vi "Main.vi"() -> ()   [LabVIEW 2021]
doc: "Use this template to build a simple state machine design pattern. Each state executes code and determines which state to transition to."
uses:
  controls/State.ctl
  controls/Data.ctl
  vmmso/vmmso.lvlib
panel:
  out "IO Read Return":u32 format="%x"
  out "IO4":bool
  out "IO0":bool
  out "Is IO Ready?":bool
  in  "DDS2 Amplitude":dbl=2000.0
  in  "DDS2 Bias":dbl
  in  "DDS2 Freq":dbl=1000.0
  in  "DDS2 Wave Style":u16(ring) items=["Sine", "Square", "Ramp"]
  in  "DDS1 Amplitude":dbl=2000.0
  in  "DDS1 Bias":dbl
  in  "DDS1 Freq":dbl=1000.0
  in  "DDS1 Wave Style":u16(ring) items=["Sine", "Square", "Ramp"]
  out "Is Data Ready？":bool
  out "ReadVoltageData Return":u32
  out "Voltage Wave":dbl[][](graph)
  out "Capture Return":i32
  out "Device is OK?":bool
  out "Support Samples":u32[](array[numeric])
  in  "Exit":bool
  # "DDS1"
  # "DDS2"
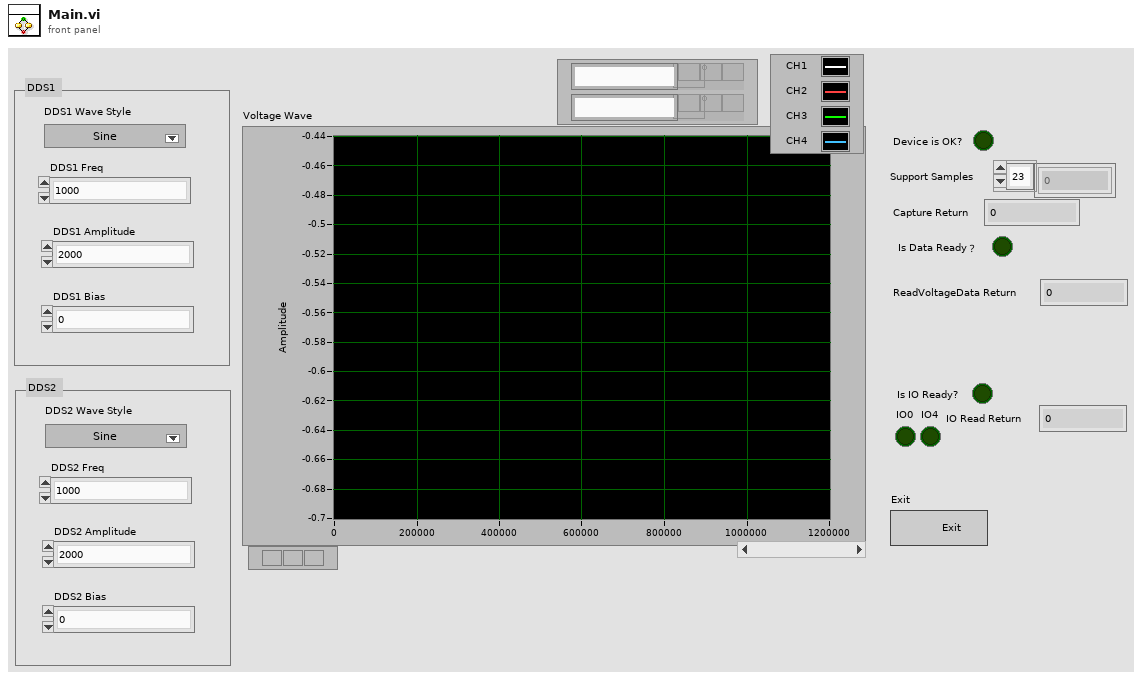
[diagram p1: front panel]
types:
  T1 = typedef "Data.ctl" = cluster{"Boolean <Is Exit>":bool, "String <Replace Me>":string, "Numeric <Replace Me>":dbl}
  T2 = typedef "State.ctl" = enum16{"Initialize", "Wait for UsbIn", "Init Osc and Dds", "Wait for Event", "Capture", "Read Voltage", "Read IO", "Exit"}
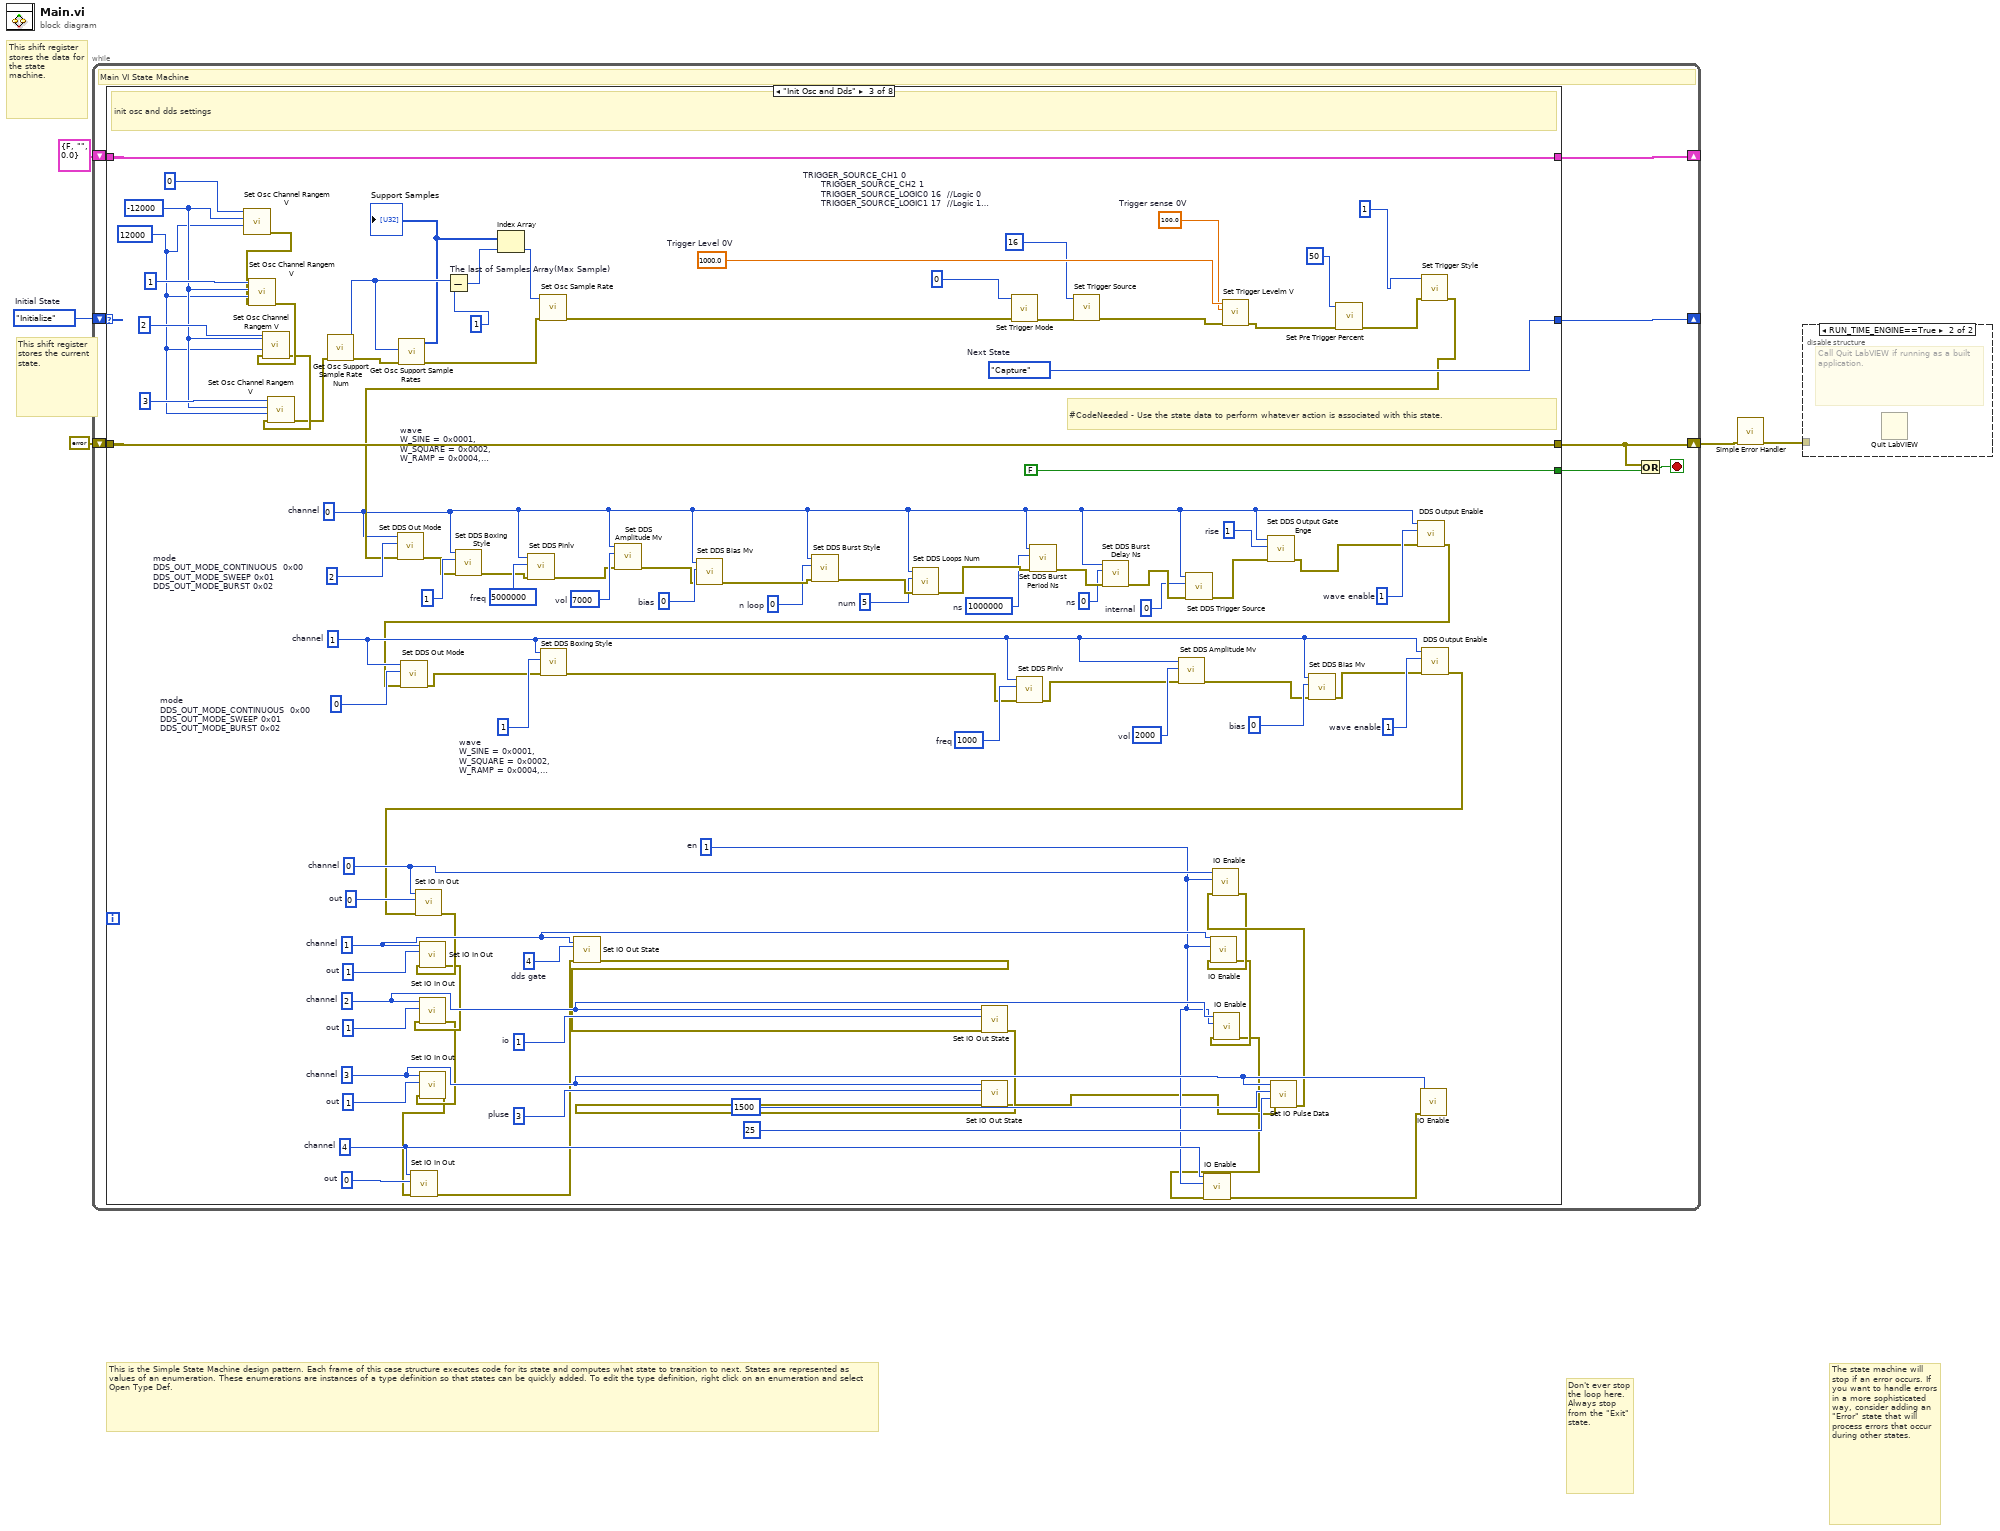
[diagram p0: block diagram]
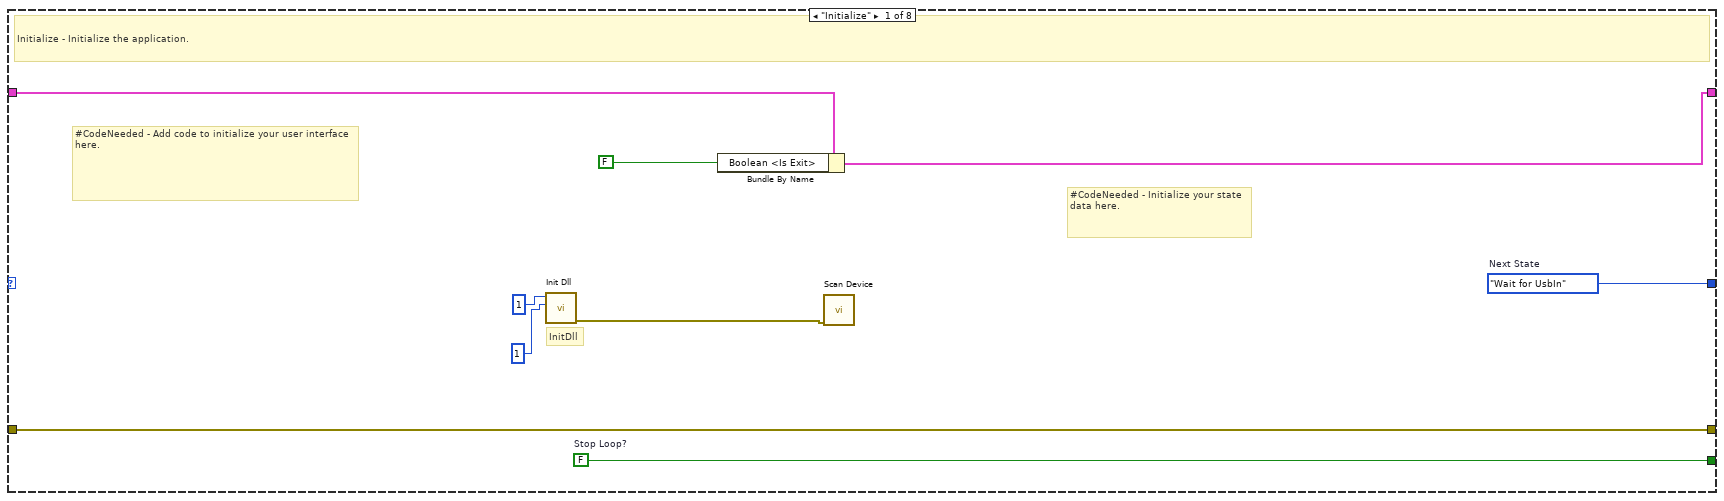
[diagram p3: hidden frame]
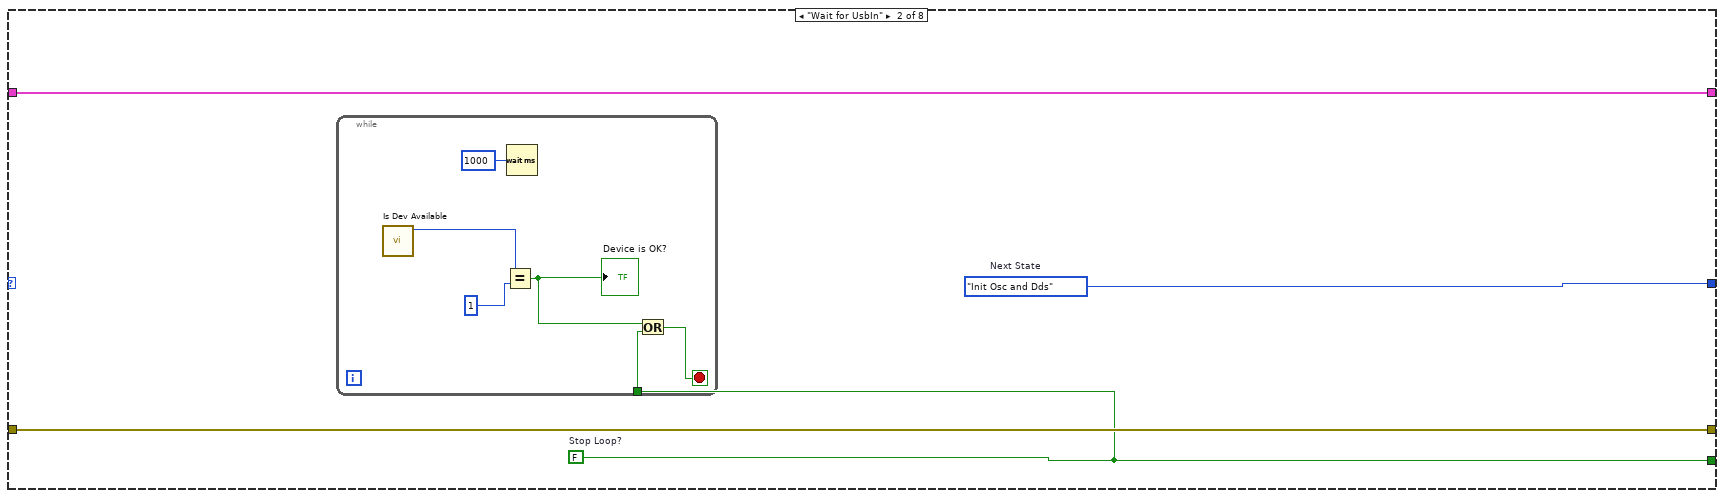
[diagram p4: hidden frame]
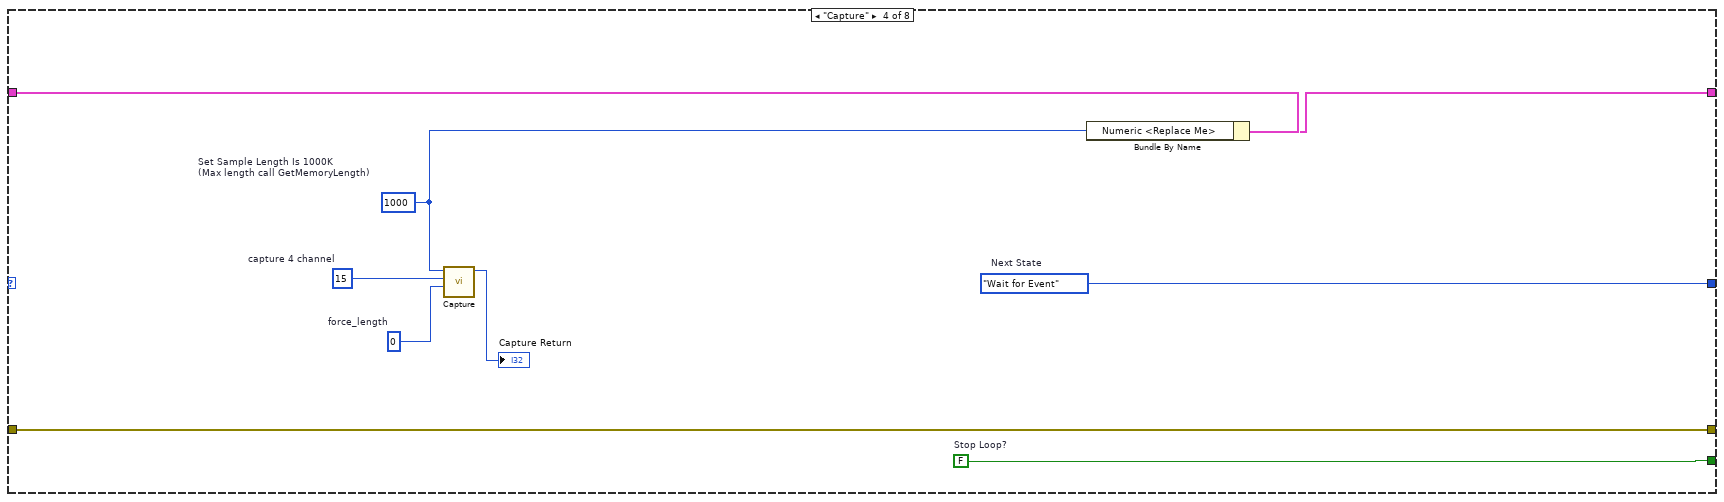
[diagram p5: hidden frame]
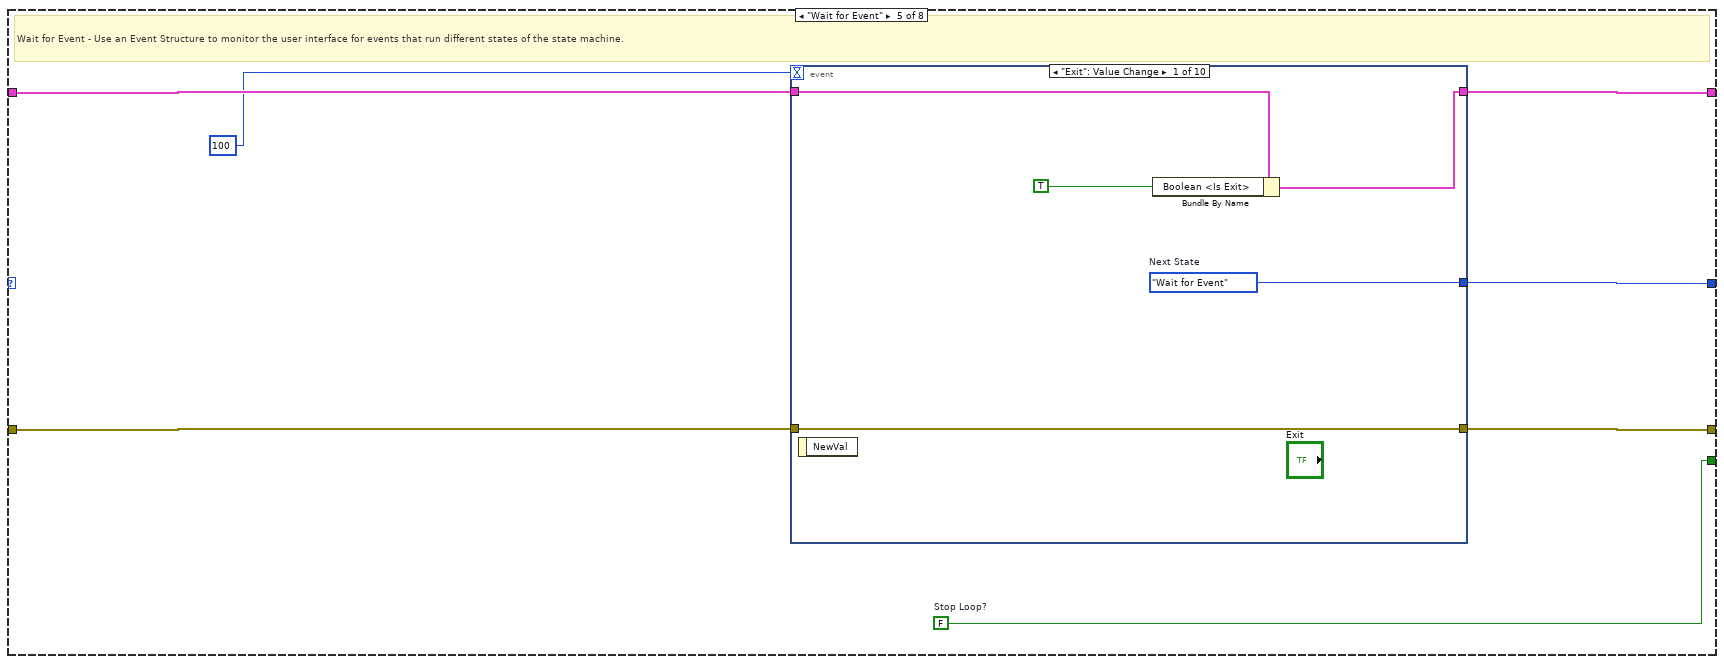
[diagram p6: hidden frame]
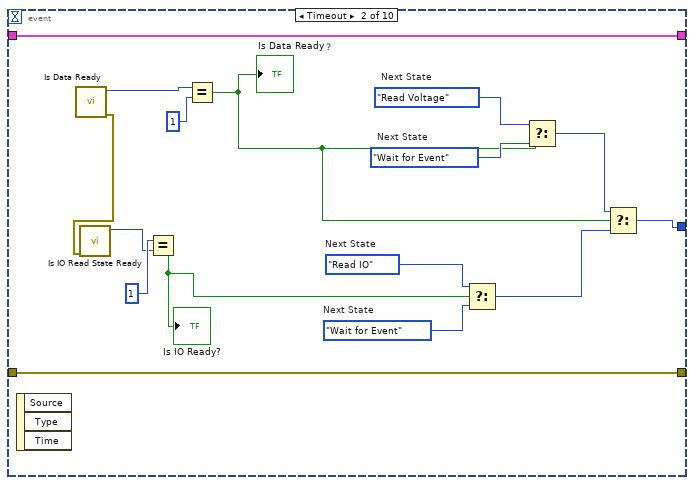
[diagram p7: hidden frame]
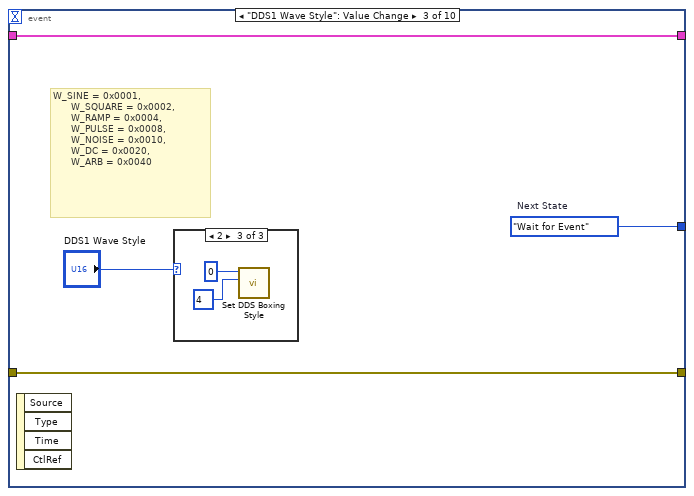
[diagram p8: hidden frame]
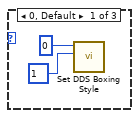
[diagram p9: hidden frame]
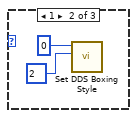
[diagram p10: hidden frame]
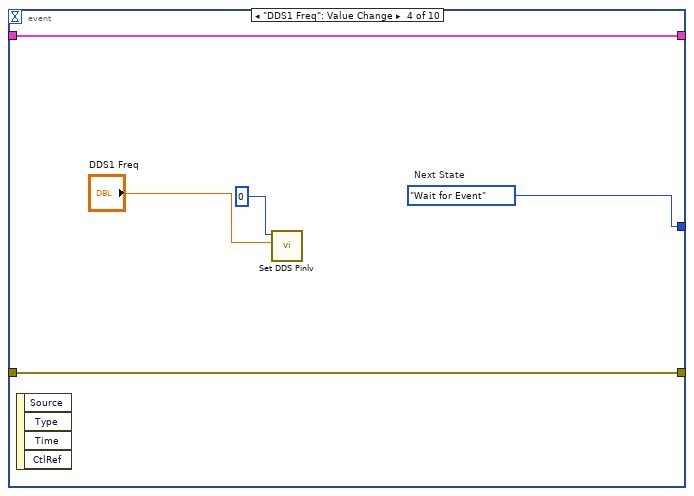
[diagram p11: hidden frame]
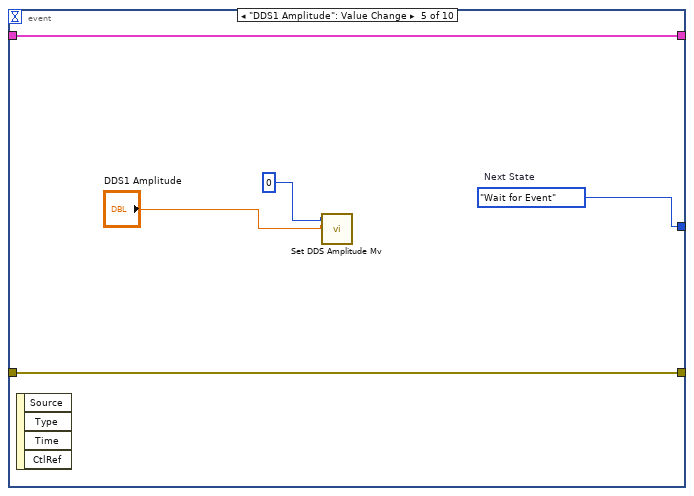
[diagram p12: hidden frame]
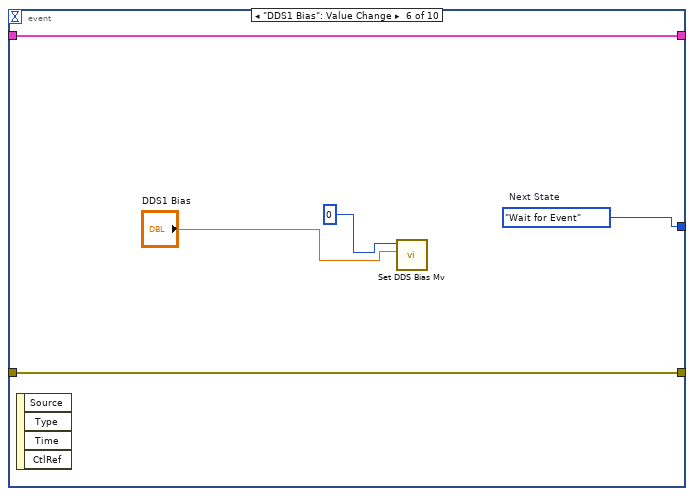
[diagram p13: hidden frame]
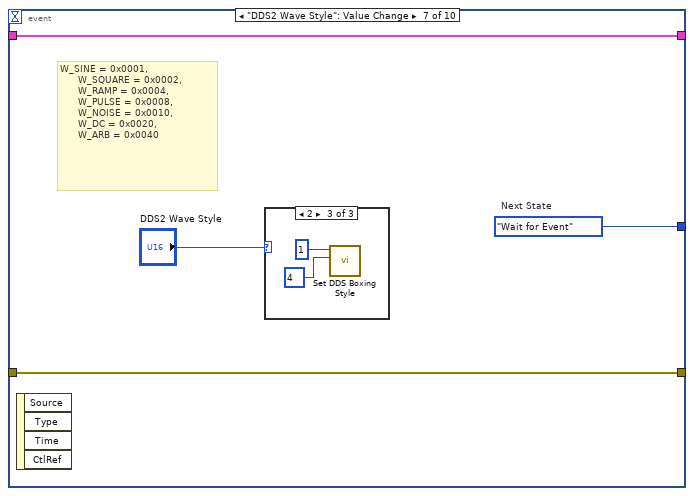
[diagram p14: hidden frame]
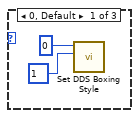
[diagram p15: hidden frame]
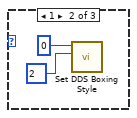
[diagram p16: hidden frame]
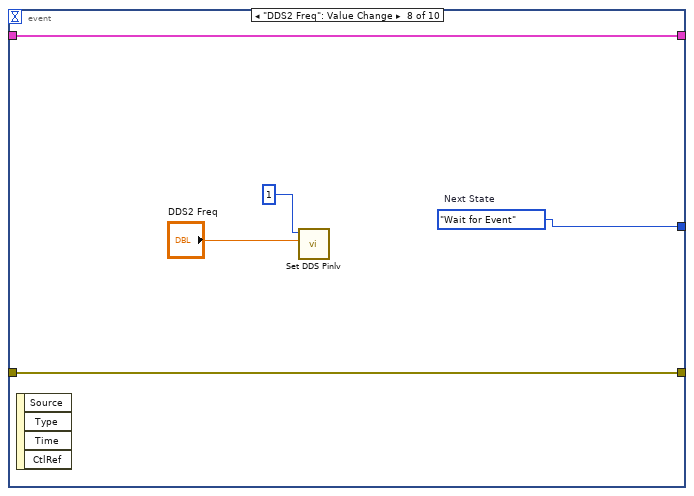
[diagram p17: hidden frame]
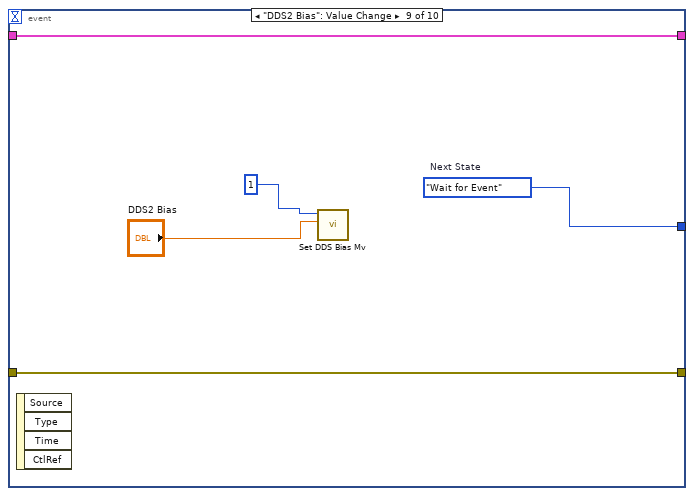
[diagram p18: hidden frame]
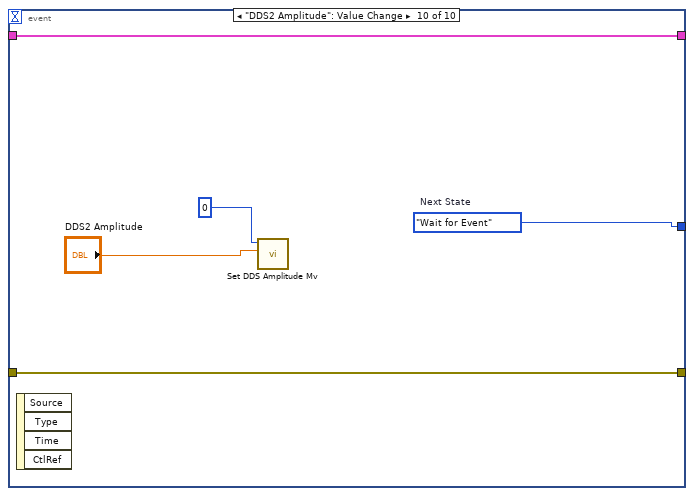
[diagram p19: hidden frame]
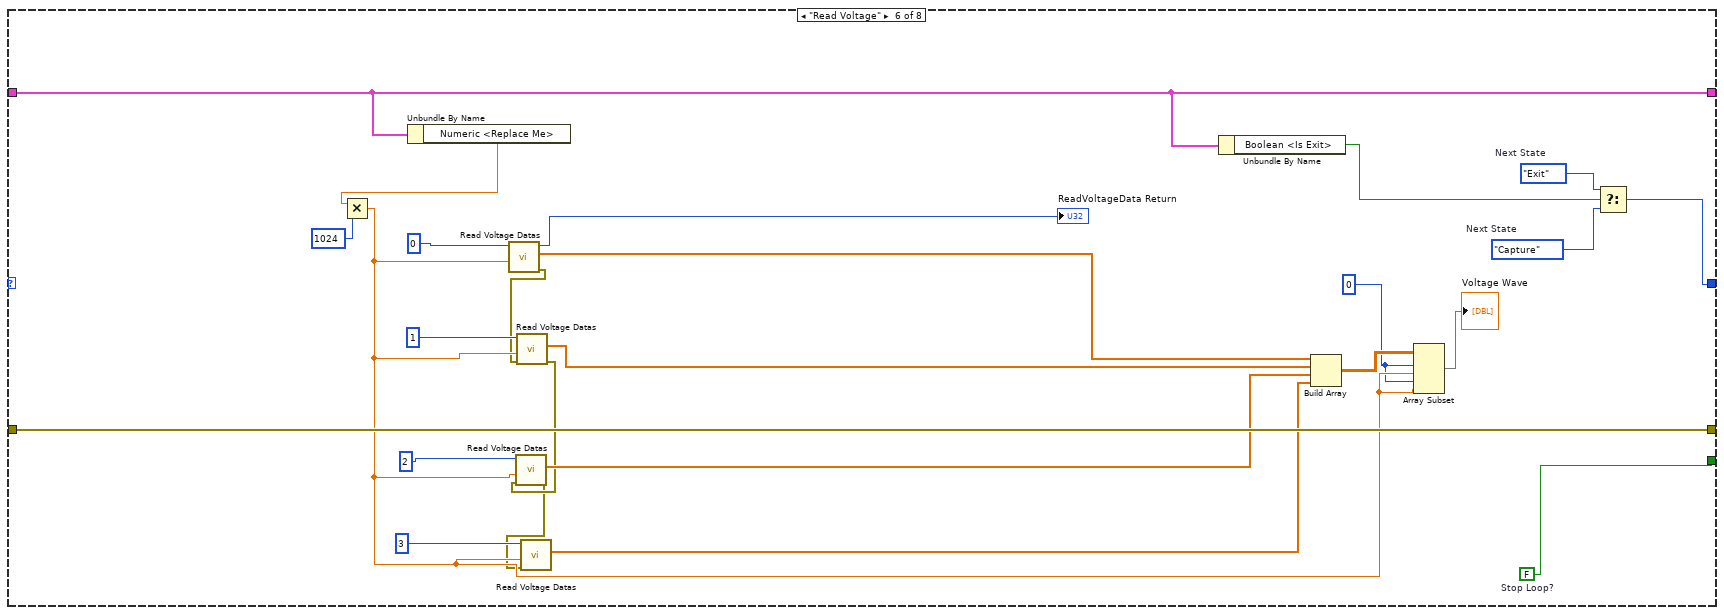
[diagram p20: hidden frame]
diagram:
  w5 = State."Initialize"  # Initial State
  # "Don't ever stop the loop here. Always stop from the \"Exit\" state."
  # "The state machine will stop if an error occurs. If you want to handle errors in a more sophisticated way, consider adding an \"Error\" state that will process errors that occur during other states."
  # "This shift register stores the data for the state machine."
  # "This is the Simple State Machine design pattern. Each frame of this case structure executes code for its state and computes what state to transition to next. States are represented as values of an enumeration. These enumerations are instances of a type definition so that states can be quickly added. To edit the type definition, right click on an enumeration and select Open Type Def."
  # "This shift register stores the current state."
  n1 = while {
    shift-right: [w12] -> _
    shift-left: w5 -> [w13]
    shift-right: [w10] -> _
    shift-left: T1 {"Boolean <Is Exit>"=FALSE, "String <Replace Me>"="", "Numeric <Replace Me>"=0.0} ("Data") -> [w11]
    shift-right: [w7] -> w2
    shift-left: errorcluster {"status"=FALSE, "code"=0, "source"=""} ("error constant") -> [w9]
    stop <- w8 stop-if-true
    # "Main VI State Machine"
    n2 = case shown="\"Init Osc and Dds\"" w13 {
      tunnel: [w22 w25 w132 w140 w148 w221 w246 w260] -> w12
      tunnel: w11 -> [w15 w23 w130 w135 w147 w224 w255 w259]
      tunnel: [w14 w23 w130 w134 w146 w224 w255 w259] -> w10
      tunnel: w9 -> [w20 w26 w129 w141 w145 w244 w254 w257]
      tunnel: [w20 w26 w129 w141 w144 w244 w254 w257] -> w7
      tunnel: [w21 w24 FALSE ("Stop Loop?") w139 w142 w243 w245 w258] -> w6
      frame "Initialize" {
        w21 = FALSE  # Stop Loop?
        w22 = State."Wait for UsbIn"  # Next State
        # "InitDll"
        # "#CodeNeeded - Initialize your state data here."
        # "#CodeNeeded - Add code to initialize your user interface here."
        # "Initialize - Initialize the application."
        n3 = call "Init Dll.vi"("en_hard_watchdog"=1 ("channel"), "en_log"=1 ("channel")) -> ("error out"=w17:errorcluster)  [unwired: 8 in, 1 out]
        n4 = Bundle By Name(cluster=w15, "Boolean <Is Exit>"=FALSE) -> (w14:T1)
        n5 = call "Scan Device.vi"("error in (no error)"=w17) -> ()  [unwired: 9 in, 2 out]
      }
      frame "Wait for UsbIn" {
        w25 = State."Init Osc and Dds"  # Next State
        w24 = FALSE  # Stop Loop?
        n6 = while {
          tunnel: w24 -> [w30]
          stop <- w29 stop-if-true
          n7 = call "Is Dev Available.vi"() -> ("function return"=w28:i32)  [unwired: 10 in, 1 out]
          n8 = Equal?(x=w28, y=1 ("channel")) -> (x = y?=w27:bool)
          "Device is OK?" <- w27
          n9 = Wait (ms)(milliseconds to wait=u32 1000 ("等待时间（毫秒）")) -> ()  [unwired: 1 out]
          n10 = Or(x=w27, y=w30) -> (x .or. y?=w29:bool)
        }
      }
      frame "Init Osc and Dds" {
        w33 = u32 1  # rise
        w37 = u32 0  # internal
        w39 = u32 0  # ns
        w41 = u32 1000000  # ns
        w43 = u32 5  # num
        w45 = u32 0  # n loop
        w85 = i8 0  # out
        w84 = i8 4  # channel
        w89 = i8 3  # pluse
        w90 = i8 1  # out
        w88 = i8 3  # channel
        w83 = i8 1  # en
        w94 = i8 4  # dds gate
        w95 = i8 1  # io
        w96 = i8 1  # out
        w91 = i8 2  # channel
        w97 = i8 1  # out
        w92 = i8 1  # channel
        w98 = i8 0  # out
        w93 = i8 0  # channel
        w99 = sgl 100.0  # Trigger sense 0V
        w106 = i8 0  # mode DDS_OUT_MODE_CONTINUOUS  0x00 DDS_OUT_MODE_SWEEP 0x01 DDS_OUT_MODE_BURST 0x02
        w108 = i8 1  # wave enable
        w110 = u32 0  # bias
        w109 = u32 2000  # vol
        w111 = u32 1000  # freq
        w112 = i8 1  # wave  W_SINE = 0x0001,  W_SQUARE = 0x0002,  W_RAMP = 0x0004,  W_PULSE = 0x0008,  W_NOISE = 0x0010,  W_DC = 0x0020,  W_ARB = 0x0040
        w107 = i8 1  # channel
        w113 = i8 2  # mode DDS_OUT_MODE_CONTINUOUS  0x00 DDS_OUT_MODE_SWEEP 0x01 DDS_OUT_MODE_BURST 0x02
        w114 = i8 1  # wave enable
        w116 = u32 0  # bias
        w115 = u32 7000  # vol
        w117 = u32 5000000  # freq
        w118 = i8 1  # wave  W_SINE = 0x0001,  W_SQUARE = 0x0002,  W_RAMP = 0x0004,  W_PULSE = 0x0008,  W_NOISE = 0x0010,  W_DC = 0x0020,  W_ARB = 0x0040
        w34 = i8 0  # channel
        w121 = 16  # TRIGGER_SOURCE_CH1 0 						TRIGGER_SOURCE_CH2 1 						TRIGGER_SOURCE_LOGIC0 16  //Logic 0 						TRIGGER_SOURCE_LOGIC1 17  //Logic 1 						TRIGGER_SOURCE_LOGIC2 18  //Logic 2 						TRIGGER_SOURCE_LOGIC3 19  //Logic 3
        w126 = sgl 1000.0  # Trigger Level 0V
        w101 = 12000 ("minmv")
        w102 = -12000 ("minmv")
        w132 = State."Capture"  # Next State
        # "#CodeNeeded - Use the state data to perform whatever action is associated with this state."
        # "init osc and dds settings"
        n11 = call "Set Osc Channel Rangem V.vi"("maxmv"=w101, "minmv"=w102, "channel"=0) -> ("error out"=w82:errorcluster)  [unwired: 7 in, 1 out]
        n12 = call "Set Osc Channel Rangem V.vi"("error in (no error)"=w82, "maxmv"=w101, "minmv"=w102, "channel"=1) -> ("error out"=w81:errorcluster)  [unwired: 6 in, 1 out]
        n13 = call "Set Osc Channel Rangem V.vi"("error in (no error)"=w81, "maxmv"=w101, "minmv"=w102, "channel"=2) -> ("error out"=w80:errorcluster)  [unwired: 6 in, 1 out]
        n14 = call "Set Osc Channel Rangem V.vi"("error in (no error)"=w80, "maxmv"=w101, "minmv"=w102, "channel"=3) -> ("error out"=w79:errorcluster)  [unwired: 6 in, 1 out]
        n15 = call "Get Osc Support Sample Rate Num.vi"("error in (no error)"=w79) -> ("error out"=w78:errorcluster, "function return"=w123:i32)  [unwired: 9 in]
        n16 = call "Get Osc Support Sample Rates.vi"("error in (no error)"=w78, "maxnum"=w123) -> ("error out"=w77:errorcluster, "sample out"=w120:u32[])  [unwired: 7 in, 1 out]
        "Support Samples" <- w120
        n17 = Subtract "The last of Samples Array(Max Sample)"(x=w123, y=1 ("front")) -> (x-y=w125:i32)
        n18 = Index Array(array=w120, index=w125) -> (element=w100:u32)
        n19 = call "Set Osc Sample Rate.vi"("error in (no error)"=w77, "sample"=w100) -> ("error out"=w76:errorcluster)  [unwired: 8 in, 1 out]
        n20 = call "Set Trigger Mode.vi"("error in (no error)"=w76, "mode"=0 ("front")) -> ("error out"=w75:errorcluster)  [unwired: 9 in]
        n21 = call "Set Trigger Source.vi"("error in (no error)"=w75, "source"=w121) -> ("error out"=w74:errorcluster)  [unwired: 9 in]
        n22 = call "Set Trigger Levelm V.vi"("error in (no error)"=w74, "sense_mv"=w99, "level_mv"=w126) -> ("error out"=w73:errorcluster)  [unwired: 8 in]
        n23 = call "Set Pre Trigger Percent.vi"("error in (no error)"=w73, "front"=50) -> ("error out"=w72:errorcluster)  [unwired: 9 in]
        n24 = call "Set Trigger Style.vi"("error in (no error)"=w72, "style"=u32 1) -> ("error out"=w71:errorcluster)  [unwired: 9 in]
        n25 = call "Set DDS Out Mode.vi"("error in (no error)"=w71, "out_mode"=w113, "channel_index"=w34) -> ("error out"=w70:errorcluster)  [unwired: 8 in]
        n26 = call "Set DDS Boxing Style.vi"("error in (no error)"=w70, "boxing"=w118, "channel_index"=w34) -> ("error out"=w69:errorcluster)  [unwired: 8 in]
        n27 = call "Set DDS Pinlv.vi"("error in (no error)"=w69, "pinlv"=w117, "channel_index"=w34) -> ("error out"=w68:errorcluster)  [unwired: 8 in]
        n28 = call "Set DDS Amplitude Mv.vi"("error in (no error)"=w68, "amplitdude"=w115, "channel_index"=w34) -> ("error out"=w67:errorcluster)  [unwired: 8 in]
        n29 = call "Set DDS Bias Mv.vi"("error in (no error)"=w67, "bias"=w116, "channel_index"=w34) -> ("error out"=w46:errorcluster)  [unwired: 8 in]
        n30 = call "Set DDS Burst Style.vi"("error in (no error)"=w46, "style"=w45, "channel_index"=w34) -> ("error out"=w44:errorcluster)  [unwired: 8 in]
        n31 = call "Set DDS Loops Num.vi"("error in (no error)"=w44, "num"=w43, "channel_index"=w34) -> ("error out"=w42:errorcluster)  [unwired: 8 in]
        n32 = call "Set DDS Burst Period Ns.vi"("error in (no error)"=w42, "ns"=w41, "channel_index"=w34) -> ("error out"=w40:errorcluster)  [unwired: 8 in]
        n33 = call "Set DDS Burst Delay Ns.vi"("error in (no error)"=w40, "ns"=w39, "channel_index"=w34) -> ("error out"=w38:errorcluster)  [unwired: 8 in]
        n34 = call "Set DDS Trigger Source.vi"("error in (no error)"=w38, "src"=w37, "channel_index"=w34) -> ("error out"=w36:errorcluster)  [unwired: 8 in]
        n35 = call "Set DDS Output Gate Enge.vi"("error in (no error)"=w36, "enge"=w33, "channel_index"=w34) -> ("error out"=w35:errorcluster)  [unwired: 8 in]
        n36 = call "DDS Output Enable.vi"("error in (no error)"=w35, "enable"=w114, "channel_index"=w34) -> ("error out"=w66:errorcluster)  [unwired: 8 in]
        n37 = call "Set DDS Out Mode.vi"("error in (no error)"=w66, "out_mode"=w106, "channel_index"=w107) -> ("error out"=w65:errorcluster)  [unwired: 8 in]
        n38 = call "Set DDS Boxing Style.vi"("error in (no error)"=w65, "boxing"=w112, "channel_index"=w107) -> ("error out"=w64:errorcluster)  [unwired: 8 in]
        n39 = call "Set DDS Pinlv.vi"("error in (no error)"=w64, "pinlv"=w111, "channel_index"=w107) -> ("error out"=w63:errorcluster)  [unwired: 8 in]
        n40 = call "Set DDS Amplitude Mv.vi"("error in (no error)"=w63, "amplitdude"=w109, "channel_index"=w107) -> ("error out"=w62:errorcluster)  [unwired: 8 in]
        n41 = call "Set DDS Bias Mv.vi"("error in (no error)"=w62, "bias"=w110, "channel_index"=w107) -> ("error out"=w61:errorcluster)  [unwired: 8 in]
        n42 = call "DDS Output Enable.vi"("error in (no error)"=w61, "enable"=w108, "channel_index"=w107) -> ("error out"=w60:errorcluster)  [unwired: 8 in]
        n43 = call "Set IO In Out.vi"("error in (no error)"=w60, "inout"=w98, "channel"=w93) -> ("error out"=w59:errorcluster)  [unwired: 8 in]
        n44 = call "Set IO In Out.vi"("error in (no error)"=w59, "inout"=w97, "channel"=w92) -> ("error out"=w58:errorcluster)  [unwired: 8 in]
        n45 = call "Set IO In Out.vi"("error in (no error)"=w58, "inout"=w96, "channel"=w91) -> ("error out"=w57:errorcluster)  [unwired: 8 in]
        n46 = call "Set IO In Out.vi"("error in (no error)"=w57, "inout"=w90, "channel"=w88) -> ("error out"=w56:errorcluster)  [unwired: 8 in]
        n47 = call "Set IO In Out.vi"("error in (no error)"=w56, "inout"=w85, "channel"=w84) -> ("error out"=w55:errorcluster)  [unwired: 8 in]
        n48 = call "Set IO Out State.vi"("error in (no error)"=w55, "state"=w94, "channel"=w92) -> ("error out"=w54:errorcluster)  [unwired: 8 in]
        n49 = call "Set IO Out State.vi"("error in (no error)"=w54, "state"=w95, "channel"=w91) -> ("error out"=w53:errorcluster)  [unwired: 8 in]
        n50 = call "Set IO Out State.vi"("error in (no error)"=w53, "state"=w89, "channel"=w88) -> ("error out"=w52:errorcluster)  [unwired: 8 in]
        n51 = call "Set IO Pulse Data.vi"("error in (no error)"=w52, "duty"=25 ("minmv"), "hz"=1500 ("minmv"), "channel"=w88) -> ("error out"=w51:errorcluster)  [unwired: 7 in]
        n52 = call "IO Enable.vi"("error in (no error)"=w51, "enable"=w83, "channel"=w93) -> ("error out"=w50:errorcluster)  [unwired: 8 in]
        n53 = call "IO Enable.vi"("error in (no error)"=w50, "enable"=w83, "channel"=w92) -> ("error out"=w49:errorcluster)  [unwired: 8 in]
        n54 = call "IO Enable.vi"("error in (no error)"=w49, "enable"=w83, "channel"=w91) -> ("error out"=w48:errorcluster)  [unwired: 8 in]
        n55 = call "IO Enable.vi"("error in (no error)"=w48, "enable"=w83, "channel"=w84) -> ("error out"=w47:errorcluster)  [unwired: 8 in]
        n56 = call "IO Enable.vi"("error in (no error)"=w47, "channel"=w88) -> ()  [unwired: 9 in, 1 out]
      }
      frame "Capture" {
        w136 = i8 0  # force_length
        w133 = u32 1000  # Set Sample Length Is 1000K (Max length call GetMemoryLength)
        w137 = i8 15  # capture 4 channel
        w139 = FALSE  # Stop Loop?
        w140 = State."Wait for Event"  # Next State
        n57 = call "Capture.vi"("force_length"=w136, "capture_channel"=w137, "length"=w133) -> ("function return"=→"Capture Return":i32)  [unwired: 7 in, 1 out]
        n58 = Bundle By Name(cluster=w135, "Numeric <Replace Me>"=w133) -> (w134:T1)
      }
      frame "Wait for Event" {
        w142 = FALSE  # Stop Loop?
        # "Wait for Event - Use an Event Structure to monitor the user interface for events that run different states of the state machine."
        n59 = event shown="[0] \"Exit\": Value Change" {
          selector: _ -> [_ _ _ _ _ _ _ _ _ _]
          dyn-events: _ -> [_ _ _ _ _ _ _ _ _ _]
          timeout: 100 ("y") -> [_ _ _ _ _ _ _ _ _ _]
          tunnel: [w153 w156 w170 w182 w187 w192 w196 w206 w211 w216] -> w148
          tunnel: w147 -> [w150 w169 w173 w184 w189 w194 w198 w209 w214 w219]
          tunnel: [w149 w169 w173 w184 w189 w194 w198 w209 w214 w219] -> w146
          tunnel: w145 -> [w152 w168 w172 w183 w188 w193 w197 w208 w213 w218]
          tunnel: [w152 w168 w172 w183 w188 w193 w197 w208 w213 w218] -> w144
          event "Exit": Value Change {
            w153 = State."Wait for Event"  # Next State
            n60 = event-data() -> ()  [unwired: 1 in, 1 out]
            n61 = Bundle By Name(cluster=w150, "Boolean <Is Exit>"=TRUE) -> (w149:T1)
          }
          event Timeout {
            w161 = State."Wait for Event"  # Next State
            w162 = State."Read IO"  # Next State
            w164 = State."Wait for Event"  # Next State
            w165 = State."Read Voltage"  # Next State
            n62 = event-data() -> ()  [unwired: 1 in, 3 out]
            n63 = call "Is Data Ready.vi"() -> ("error out"=w154:errorcluster, "function return"=w167:i32)  [unwired: 10 in]
            n64 = call "Is IO Read State Ready.vi"("error in (no error)"=w154) -> ("function return"=w155:i32)  [unwired: 9 in, 1 out]
            n65 = Equal?(x=1 ("y"), y=w155) -> (x = y?=w163:bool)
            "Is IO Ready?" <- w163
            n66 = Equal?(x=w167, y=1) -> (x = y?=w157:bool)
            "Is Data Ready？" <- w157
            n67 = Select(t=w162, s=w163, f=w161) -> (s? t:f=w159:T2)
            n68 = Select(t=w165, s=w157, f=w164) -> (s? t:f=w158:T2)
            n69 = Select(t=w158, s=w157, f=w159) -> (s? t:f=w156:T2)
          }
          event "DDS1 Wave Style": Value Change {
            w170 = State."Wait for Event"  # Next State
            # "W_SINE = 0x0001, \n\t\t\t\t\t\tW_SQUARE = 0x0002, \n\t\t\t\t\t\tW_RAMP = 0x0004, \n\t\t\t\t\t\tW_PULSE = 0x0008, \n\t\t\t\t\t\tW_NOISE = 0x0010, \n\t\t\t\t\t\tW_DC = 0x0020, \n\t\t\t\t\t\tW_ARB = 0x0040"
            n70 = event-data() -> ()  [unwired: 1 in, 4 out]
            n71 = case shown="2" "DDS1 Wave Style" {
              frame 0, Default {
                n72 = call "Set DDS Boxing Style.vi"("boxing"=1 ("y"), "channel_index"=0 ("y")) -> ()  [unwired: 9 in, 1 out]
              }
              frame 1 {
                n73 = call "Set DDS Boxing Style.vi"("boxing"=2 ("y"), "channel_index"=0 ("y")) -> ()  [unwired: 9 in, 1 out]
              }
              frame 2 {
                n74 = call "Set DDS Boxing Style.vi"("boxing"=4 ("y"), "channel_index"=0 ("y")) -> ()  [unwired: 9 in, 1 out]
              }
            }
          }
          event "DDS1 Freq": Value Change {
            w182 = State."Wait for Event"  # Next State
            n75 = event-data() -> ()  [unwired: 1 in, 4 out]
            n76 = call "Set DDS Pinlv.vi"("pinlv"="DDS1 Freq", "channel_index"=0 ("y")) -> ()  [unwired: 9 in, 1 out]
          }
          event "DDS1 Amplitude": Value Change {
            w187 = State."Wait for Event"  # Next State
            n77 = event-data() -> ()  [unwired: 1 in, 4 out]
            n78 = call "Set DDS Amplitude Mv.vi"("amplitdude"="DDS1 Amplitude", "channel_index"=0 ("y")) -> ()  [unwired: 9 in, 1 out]
          }
          event "DDS1 Bias": Value Change {
            w192 = State."Wait for Event"  # Next State
            n79 = event-data() -> ()  [unwired: 1 in, 4 out]
            n80 = call "Set DDS Bias Mv.vi"("bias"="DDS1 Bias", "channel_index"=0 ("y")) -> ()  [unwired: 9 in, 1 out]
          }
          event "DDS2 Wave Style": Value Change {
            w196 = State."Wait for Event"  # Next State
            # "W_SINE = 0x0001, \n\t\t\t\t\t\tW_SQUARE = 0x0002, \n\t\t\t\t\t\tW_RAMP = 0x0004, \n\t\t\t\t\t\tW_PULSE = 0x0008, \n\t\t\t\t\t\tW_NOISE = 0x0010, \n\t\t\t\t\t\tW_DC = 0x0020, \n\t\t\t\t\t\tW_ARB = 0x0040"
            n81 = event-data() -> ()  [unwired: 1 in, 4 out]
            n82 = case shown="2" "DDS2 Wave Style" {
              frame 0, Default {
                n83 = call "Set DDS Boxing Style.vi"("boxing"=1 ("y"), "channel_index"=0 ("y")) -> ()  [unwired: 9 in, 1 out]
              }
              frame 1 {
                n84 = call "Set DDS Boxing Style.vi"("boxing"=2 ("y"), "channel_index"=0 ("y")) -> ()  [unwired: 9 in, 1 out]
              }
              frame 2 {
                n85 = call "Set DDS Boxing Style.vi"("boxing"=4 ("y"), "channel_index"=1 ("y")) -> ()  [unwired: 9 in, 1 out]
              }
            }
          }
          event "DDS2 Freq": Value Change {
            w206 = State."Wait for Event"  # Next State
            n86 = event-data() -> ()  [unwired: 1 in, 4 out]
            n87 = call "Set DDS Pinlv.vi"("pinlv"="DDS2 Freq", "channel_index"=1 ("y")) -> ()  [unwired: 9 in, 1 out]
          }
          event "DDS2 Bias": Value Change {
            w211 = State."Wait for Event"  # Next State
            n88 = event-data() -> ()  [unwired: 1 in, 4 out]
            n89 = call "Set DDS Bias Mv.vi"("bias"="DDS2 Bias", "channel_index"=1 ("y")) -> ()  [unwired: 9 in, 1 out]
          }
          event "DDS2 Amplitude": Value Change {
            w216 = State."Wait for Event"  # Next State
            n90 = event-data() -> ()  [unwired: 1 in, 4 out]
            n91 = call "Set DDS Amplitude Mv.vi"("amplitdude"="DDS2 Amplitude", "channel_index"=0 ("y")) -> ()  [unwired: 9 in, 1 out]
          }
        }
      }
      frame "Read Voltage" {
        w223 = State."Exit"  # Next State
        w222 = State."Capture"  # Next State
        w230 = i8 0 ("channel")
        w243 = FALSE  # Stop Loop?
        n92 = Unbundle By Name(w224) -> ("Numeric <Replace Me>"=w239:dbl)
        n93 = Multiply(x=w239, y=1024) -> (x*y=w231:dbl)
        n94 = call "Read Voltage Datas.vi"("length"=w231, "channel"=i8 0) -> ("error out"=w227:errorcluster, "buffer out"=w228:dbl[], "function return"=→"ReadVoltageData Return":u32)  [unwired: 7 in]
        n95 = call "Read Voltage Datas.vi"("error in (no error)"=w227, "length"=w231, "channel"=i8 1) -> ("error out"=w226:errorcluster, "buffer out"=w235:dbl[])  [unwired: 6 in, 1 out]
        n96 = call "Read Voltage Datas.vi"("error in (no error)"=w226, "length"=w231, "channel"=i8 2) -> ("error out"=w225:errorcluster, "buffer out"=w234:dbl[])  [unwired: 6 in, 1 out]
        n97 = call "Read Voltage Datas.vi"("error in (no error)"=w225, "length"=w231, "channel"=i8 3) -> ("buffer out"=w233:dbl[])  [unwired: 6 in, 2 out]
        n98 = Unbundle By Name(w224) -> ("Boolean <Is Exit>"=w220:bool)
        n99 = Build Array(w228, w235, w234, w233) -> (w232:dbl[][])
        n100 = Array Subset(array=w232, index (row)=w230, length (row)=w231, index (col)=w230, length (col)=w231) -> (→"Voltage Wave":dbl[][])
        n101 = Select(t=w223, s=w220, f=w222) -> (s? t:f=w221:T2)
      }
      frame "Read IO" {
        w245 = FALSE  # Stop Loop?
        w246 = State."Wait for Event"  # Next State
        w252 = 16 ("front")
        w249 = 1 ("front")
        n102 = call "Get IO In State.vi"() -> ("function return"=w248:u32)  [unwired: 10 in, 1 out]
        "IO Read Return" <- w248
        n103 = And(x=w248, y=w252) -> (x .and. y?=w251:u32)
        n104 = And(x=w248, y=w249) -> (x .and. y?=w247:u32)
        n105 = Equal?(x=w247, y=w249) -> (x = y?=→"IO0":bool)
        n106 = Equal?(x=w251, y=w252) -> (x = y?=→"IO4":bool)
      }
      frame "Exit" {
        w258 = TRUE  # Stop Loop?
        w260 = State."Exit"  # (Value Not Used)
        # "#CodeNeeded - Add any required cleanup code here."
        # "The state value is not used here since this is the last iteration of the state machine loop."
        # "Exit - Exit the application."
        n107 = flat-sequence {
          tunnel: [w262] -> w256
          tunnel: w256 -> [w269]
          frame #0 {
            w263 = i8 16  # IO Num
            w262 = i8 0  # en
            n108 = for {
              N: w263 -> [_]
              tunnel: w262 -> [w266]
              i -> [w267]
              n109 = feedback #1() -> (w264:errorcluster)  [unwired: 1 in]
              n110 = call "IO Enable.vi"("error in (no error)"=w264, "enable"=w266, "channel"=w267) -> ("error out"=w265:errorcluster)  [unwired: 8 in]
              n111 = feedback-in #1(w265) -> ()
            }
            n112 = Wait (ms)(milliseconds to wait=1000) -> ()  [unwired: 1 out]
          }
          frame #1 {
            w271 = i8 1  # channel
            w270 = i8 0  # channel
            n113 = call "DDS Output Enable.vi"("enable"=w269, "channel_index"=w270) -> ("error out"=w272:errorcluster)  [unwired: 9 in]
            n114 = call "DDS Output Enable.vi"("error in (no error)"=w272, "enable"=w269, "channel_index"=w271) -> ()  [unwired: 8 in, 1 out]
            n115 = Wait (ms)(milliseconds to wait=1000) -> ()  [unwired: 1 out]
          }
          frame #2 {
            n116 = call "Finish Dll.vi"() -> ()  [unwired: 10 in, 2 out]
          }
        }
      }
    }
    n117 = Or(x=w7, y=w6) -> (x .or. y?=w8:bool)
  }
  n118 = call <vilib>:"Simple Error Handler.vi"("error in (no error)"=w2) -> ("error out"=w1:errorcluster)  [unwired: 4 in, 4 out]
  n119 = disable-structure shown="RUN_TIME_ENGINE==True" {
    disable-tunnel: w1 -> [_ _]
    frame condition #0 (active) {
    }
    frame condition #1 {
      # "Call Quit LabVIEW if running as a built application."
      n120 = Quit LabVIEW() -> ()  [unwired: 1 in]
    }
  }
